vi "Message Get Module Address.vi"(0 "Module":string) -> (1 "Address":string, 2 "Port":u16=65535)   [LabVIEW 2009]
uses:
  Message Address Global.vi
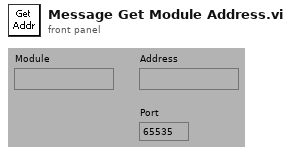
[diagram p1: front panel]
types:
  T1 = cluster{"Module":string, "Address":string, "Port":u16}[]
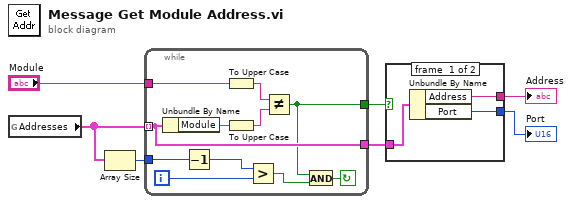
[diagram p0: block diagram]
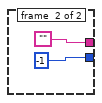
[diagram p2: hidden frame]
diagram:
  n1 = global read "Message Address Global.vi" "Addresses"() -> (w6:T1)
  n2 = Array Size(array=w6) -> (size(s)=w5:i32)
  n3 = while {
    tunnel: [w9] -> w4
    tunnel: [w10] -> w3
    tunnel: w5 -> [w14]
    tunnel: "Module" -> [w17]
    tunnel: w6 -> [w10] mode=indexing
    i -> [w13]
    stop <- w12 continue-if-true
    n4 = Unbundle By Name(w10) -> ("Module"=w18:string)
    n5 = Decrement(x=w14) -> (x-1=w8:i32)
    n6 = To Upper Case(1:w17) -> (0:w16:string)
    n7 = To Upper Case(1:w18) -> (0:w15:string)
    n8 = Greater?(x=w8, y=w13) -> (0:w11:bool)
    n9 = Not Equal?(x=w16, y=w15) -> (x != y?=w9:bool)
    n10 = And(x=w9, y=w11) -> (x .and. y?=w12:bool)
  }
  n11 = case shown="True" w4 {
    tunnel: [w21 ""] -> w2
    tunnel: [w20 -1] -> w1
    tunnel: w3 -> [w19 _]
    frame #0 {
      n12 = Unbundle By Name(w19) -> ("Address"=w21:string, "Port"=w20:u16)
    }
    frame #1 {
    }
  }
  "Address" <- w2
  "Port" <- w1
